vi "Temperhum-ManualBuilder.vi"() -> ()   [LabVIEW 2019]
uses:
  <userlib>/LevyLab/Build Support/PostBuildSupport/PostBuildSupport.lvclass
  <vilib>/MakerHub/Toolbox/LMH-Toolbox.lvlib
panel:
  in  "Package Version":string="1.0.0.8"
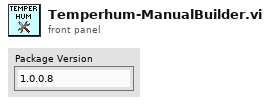
[diagram p1: front panel]
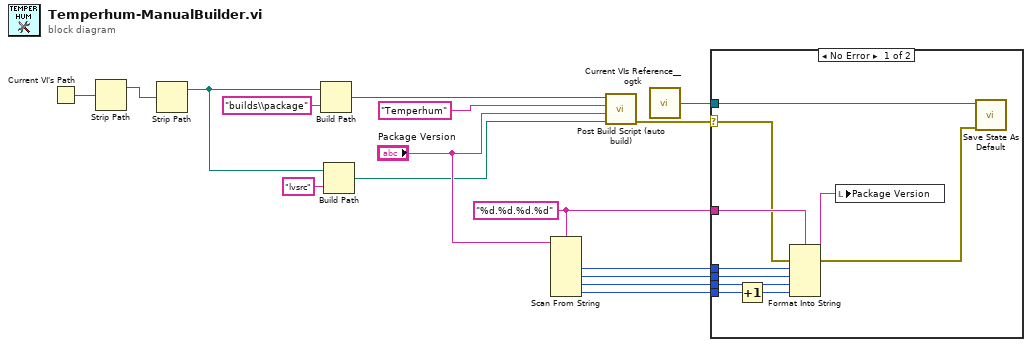
[diagram p0: block diagram]
diagram:
  w10 = "%d.%d.%d.%d" ("format string")
  n1 = Current VI's Path() -> (path=w16:path)
  n2 = Strip Path(path=w16) -> (stripped path=w15:path)  [unwired: 1 out]
  n3 = Strip Path(path=w15) -> (stripped path=w14:path)  [unwired: 1 out]
  n4 = Build Path(base path=w14, name or relative path="builds\\package") -> (appended path=w3:path)
  n5 = Build Path(base path=w14, name or relative path="lvsrc") -> (appended path=w2:path)
  n6 = Scan From String(format string=w10, input string="Package Version") -> (output 1=w9:i32, output 2=w7:i32, output 3=w8:i32, output 4=w11:i32)  [unwired: 6 in, 3 out]
  n7 = call <userlib>:"Post Build Script (auto build).vi"("Package Source Folder"=w2, "Package Version"="Package Version", "Product Name"="Temperhum", "Output Package File Path"=w3) -> ("error out"=w12:errorcluster)  [unwired: 7 in]
  n8 = call <userlib>:"Current VIs Reference__ogtk.vi"() -> ("Current VI's reference"=w6:refnum<vi>)  [unwired: 5 in]
  n9 = case shown="No Error" w12 {
    selector: w12 -> [w19 _]
    tunnel: w11 -> [w26 _]
    tunnel: w10 -> [w25 _]
    tunnel: w9 -> [w24 _]
    tunnel: w8 -> [w21 _]
    tunnel: w7 -> [w20 _]
    tunnel: w6 -> [w17 _]
    frame No Error {
      n10 = Increment(x=w26) -> (x+1=w22:i32)
      n11 = Format Into String(format string=w25, error in=w19, w24, w20, w21, w22) -> (resulting string=w23:string, error out=w18:errorcluster)  [unwired: 1 in]
      n12 = local write "Package Version"(w23) -> ()
      n13 = call <vilib>:"Save State As Default.vi"("Error In"=w18, "Target VI"=w17) -> ()  [unwired: 8 in, 2 out]
    }
    frame Error {
    }
  }
